vi "RecorderInit.vi"(4 "Number Of Motors":u8, 5 "Enable Writer":bool, 6 "Autonomous File":string, 7 "NXT":T1={"Hardware"="NXT", "Flattened String"=""}) -> (3 "NXT":T1={"Hardware"="NXT", "Flattened String"=""})   [LabVIEW 2010, in "Recorder.lvlib"]
uses:
  Recorder.lvlib
  <vilib>/NXT/Subs/LVHSConnector.ctl
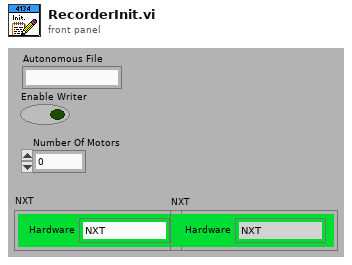
[diagram p1: front panel]
types:
  T1 = typedef "LVHSConnector.ctl" = cluster{"Hardware":string, "Flattened String":string}
  T2 = cluster{"FileName":string, "WriterEnabled?":bool, "TeleopEnabled?":bool, "StopProgram?":bool, "ArraySize":u8}
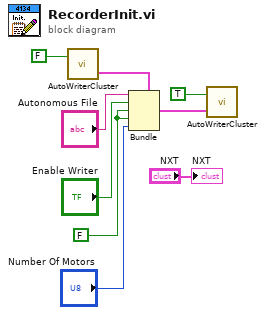
[diagram p0: block diagram]
diagram:
  w2 = FALSE
  n1 = call "AutoWriterCluster.vi"("Mode(Write=True)"=FALSE) -> ("Output"=w7:T2)  [unwired: 1 in]
  n2 = Bundle(cluster=w7, "FileName"="Autonomous File", "WriterEnabled?"="Enable Writer", "TeleopEnabled?"=w2, "StopProgram?"=w2, "ArraySize"="Number Of Motors") -> (w6:T2)
  n3 = call "AutoWriterCluster.vi"("Mode(Write=True)"=TRUE, "Input"=w6) -> ()  [unwired: 1 out]
  "NXT" <- "NXT"
